vi "TestForADP.vi"() -> ()   [LabVIEW 2019]
uses:
  <vilib>/Instr/_visa.llb/VISA Configure Serial Port (Instr).vi
  <vilib>/Utility/file.llb/Write Delimited Spreadsheet (string).vi
  <vilib>/Utility/file.llb/Write Delimited Spreadsheet (DBL).vi
  <vilib>/ptbypt/NI_PtbyPt.lvlib
panel:
  out "Present (s)":dbl
  out "Elapsed Time (s)":dbl
  out "Water Warning":bool
  out "Water Alarm":bool
  out "Water Level":dbl
  out "UV Warning":bool
  out "UV Alarm":bool
  out "UV Value":dbl
  out "Lux Chart":dbl(graph)
  out "Lux Alarm":bool
  out "Lux Warning":bool
  out "Lux Value":dbl
  out "Data: Time, Humidity, Temperature, UV, Lux, Water Level":dbl[][](array[numeric])
  in  "Temp Bias":dbl
  out "Temp. Mean":dbl format="%0.2f"
  out "Temp Chart":dbl(graph)
  out "Temp Alarm":bool
  out "Temp Warning":bool
  out "Temperature (F)":dbl
  out "Humidity Chart":dbl(graph)
  out "Humid Alarm":bool
  out "Humid Warning":bool
  out "Humidity":dbl
  out "Arduino Power":bool
  in  "Operational Mode":bool
  in  "Arduino COM Port":refnum<visa-resource-name>="COM3"
  in  "?":bool
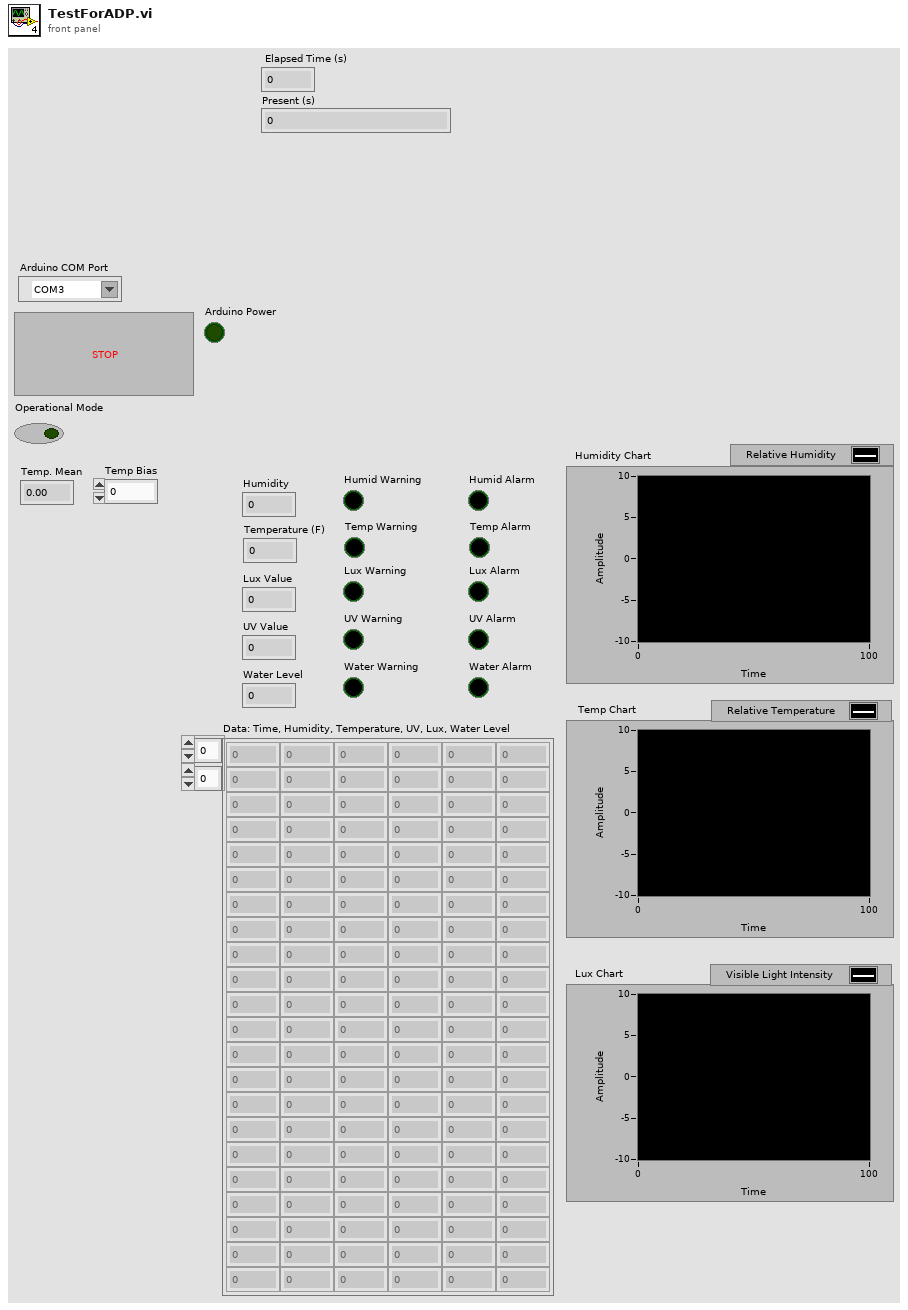
[diagram p1: front panel]
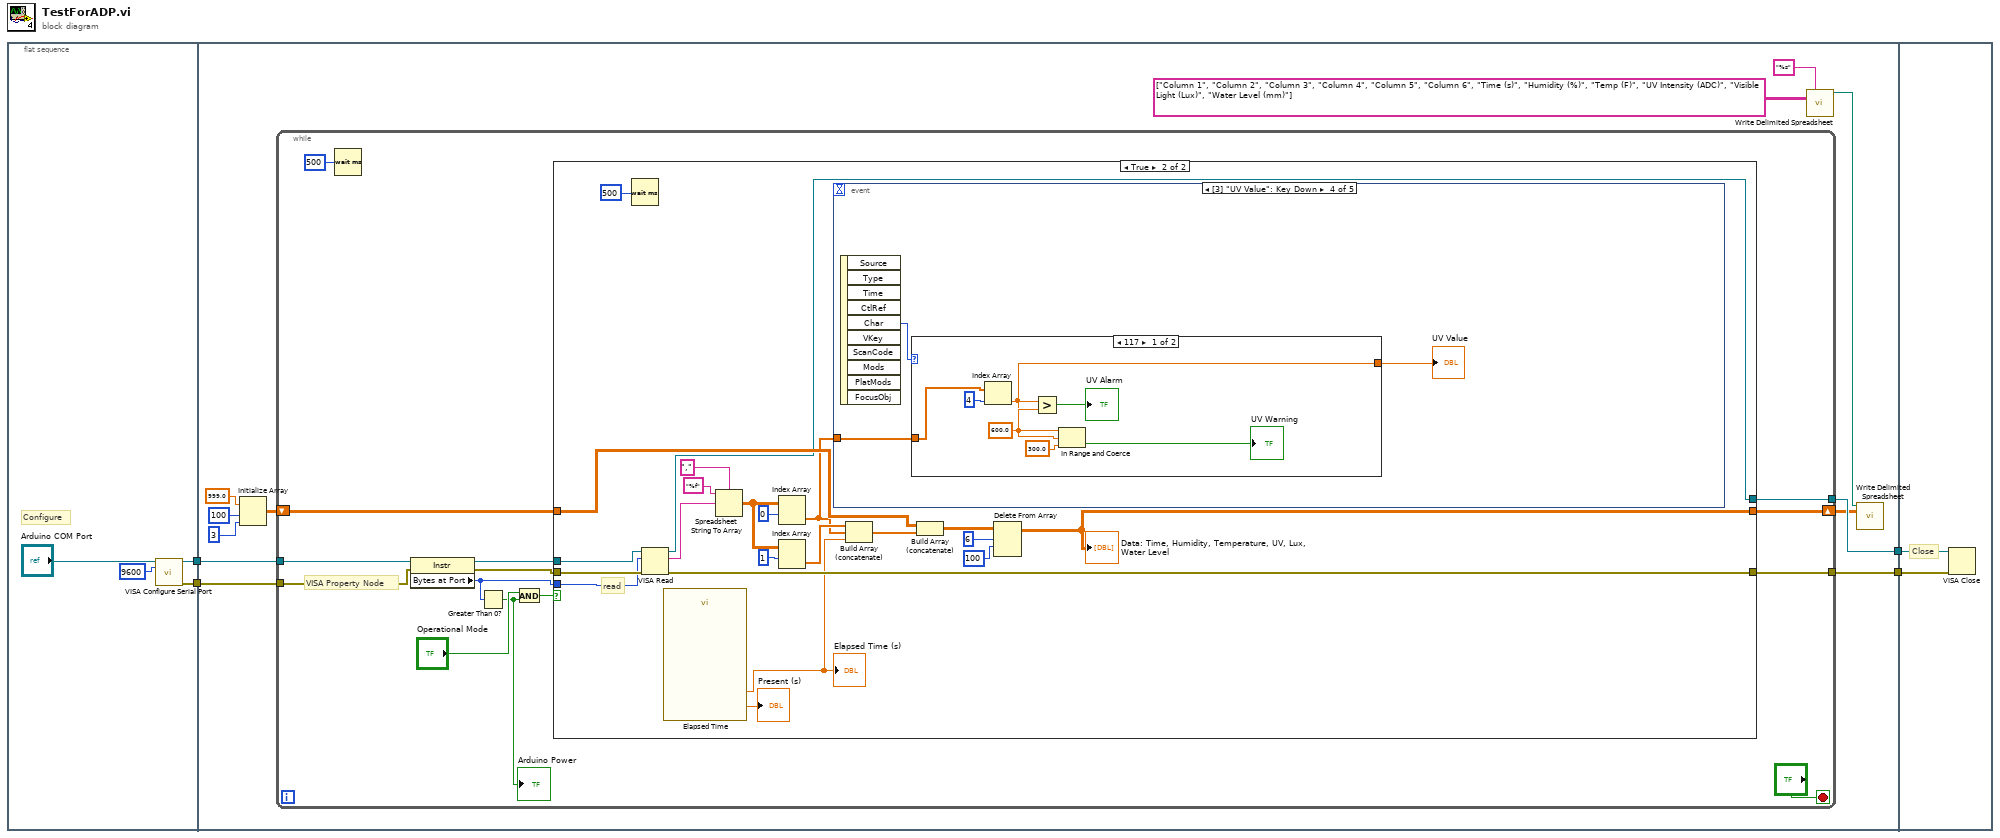
[diagram p0: block diagram]
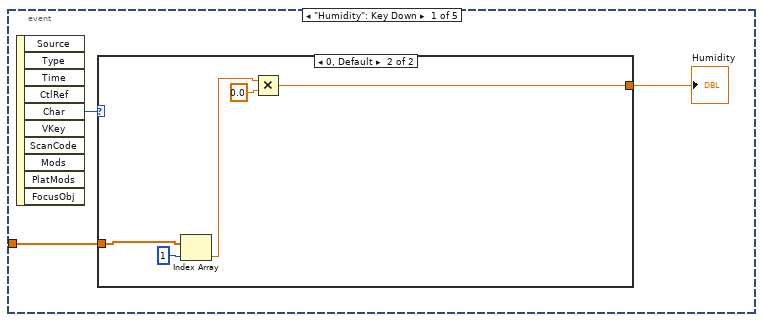
[diagram p3: hidden frame]
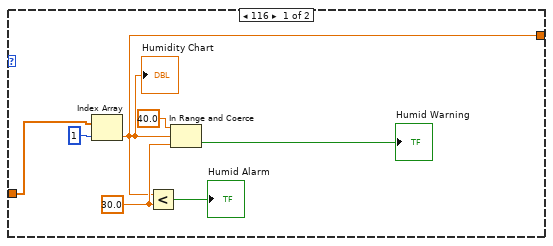
[diagram p4: hidden frame]
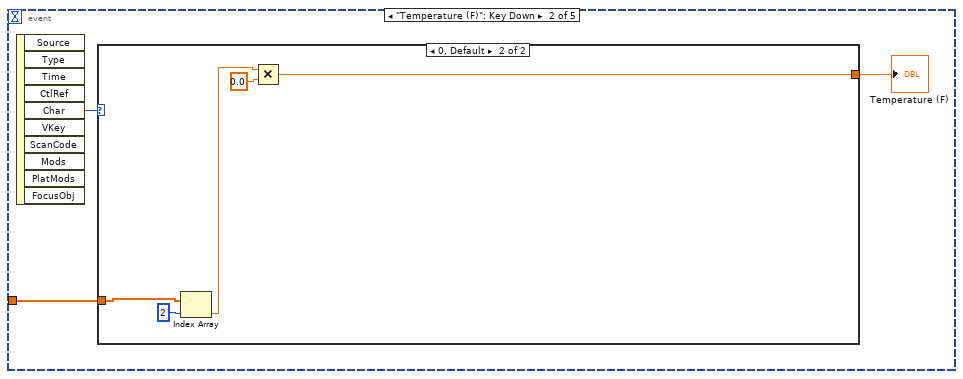
[diagram p5: hidden frame]
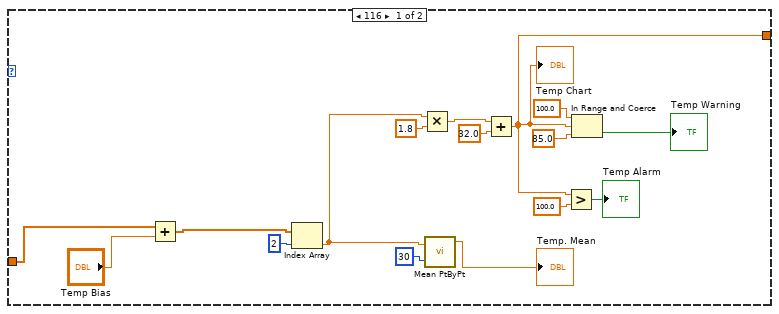
[diagram p6: hidden frame]
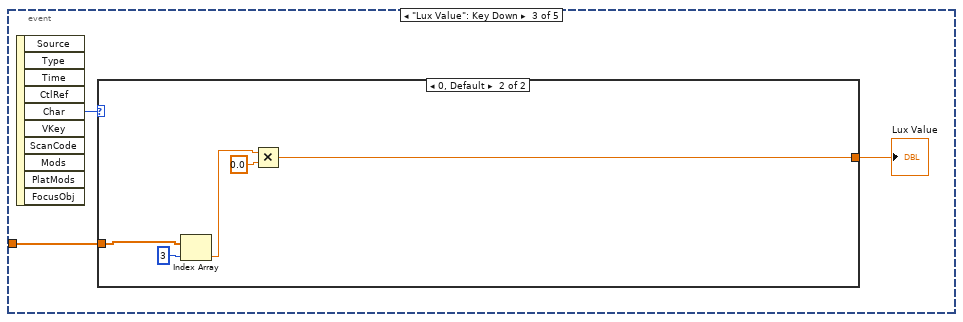
[diagram p7: hidden frame]
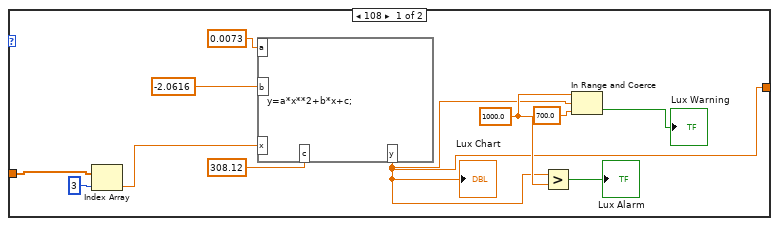
[diagram p8: hidden frame]
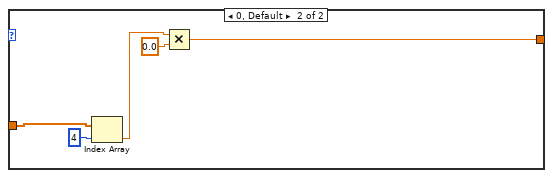
[diagram p9: hidden frame]
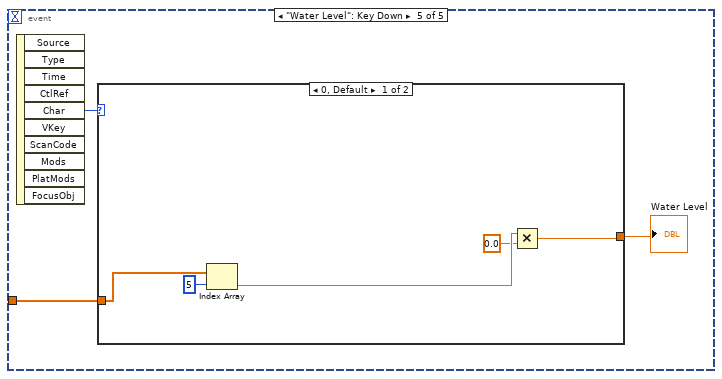
[diagram p10: hidden frame]
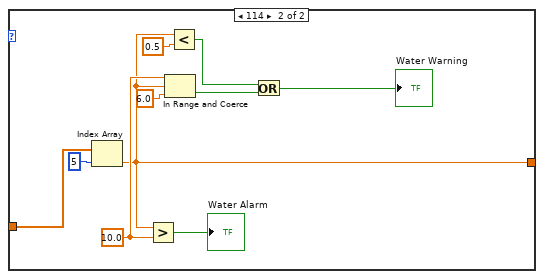
[diagram p11: hidden frame]
diagram:
  n1 = flat-sequence {
    tunnel: [w5] -> w4
    tunnel: [w6] -> w3
    tunnel: w4 -> [w20]
    tunnel: [w19] -> w2
    tunnel: w3 -> [w18]
    tunnel: [w17] -> w1
    tunnel: w2 -> [w152]
    tunnel: w1 -> [w151]
    frame #0 {
      # "Configure"
      n2 = call-poly "VISA Configure Serial Port"("VISA resource name"="Arduino COM Port", "baud rate (9600)"=u32 9600) -> ("VISA resource name out"=w5:refnum<visa-resource-name>, "error out"=w6:errorcluster)  [unwired: 12 in]
    }
    frame #1 {
      n3 = Initialize Array(999.0 ("element"), 100 ("dimension size"), 3 ("dimension size")) -> (w13:dbl[][])
      n4 = while {
        tunnel: w20 -> [w31]
        tunnel: [w23] -> w19
        tunnel: w18 -> [w30]
        tunnel: [w24] -> w17
        shift-right: [w22] -> w9
        shift-left: w13 -> [w26]
        stop <- "?" stop-if-true
        # "VISA Property Node"
        n5 = Wait (ms)(milliseconds to wait=u32 500) -> ()  [unwired: 1 out]
        n6 = property class="Instr"(reference=w31, error in=w30) -> (reference out=w28:refnum<visa-resource-name>, error out=w29:errorcluster, "Bytes at Port"=w27:u32)
        n7 = Greater Than 0?(x=w27) -> (x > 0?=w32:bool)
        "Arduino Power" <- w32
        n8 = And(x="Operational Mode", y=w32) -> (x .and. y?=w21:bool)
        n9 = case shown="True" w21 {
          tunnel: w29 -> [w36 w59]
          tunnel: w28 -> [w35 w57]
          tunnel: w27 -> [_ w58]
          tunnel: w26 -> [w37 w48]
          tunnel: [w36 w45] -> w24
          tunnel: [w35 w44] -> w23
          tunnel: [w37 w40] -> w22
          frame False {
          }
          frame True {
            # "read"
            n10 = Wait (ms)(milliseconds to wait=u32 500) -> ()  [unwired: 1 out]
            n11 = VISA Read(VISA resource name=w57, byte count=w58, error in (no error)=w59) -> (VISA resource name out=w44:refnum<visa-resource-name>, read buffer=w56:string, error out=w45:errorcluster)  [unwired: 1 out]
            n12 = call "Elapsed Time"() -> ("Present (s)"=→"Present (s)":dbl, "Elapsed Time (s)"=w39:dbl)  [unwired: 12 in, 6 out]
            "Elapsed Time (s)" <- w39
            n13 = Spreadsheet String To Array(delimiter (Tab)=",", format string="%f", spreadsheet string=w56) -> (array=w53:dbl[][])  [unwired: 1 in]
            n14 = Index Array(array=w53, index (row)=0) -> (element=w47:dbl[])  [unwired: 1 in]
            n15 = Index Array(array=w53, index (row)=1) -> (element=w50:dbl[])  [unwired: 1 in]
            n16 = event shown="[3] \"UV Value\": Key Down" {
              selector: _ -> [_ _ _ _ _]
              dyn-events: _ -> [_ _ _ _ _]
              timeout: _ -> [_ _ _ _ _]
              tunnel: w47 -> [w61 w77 w101 w120 w135]
              event "Humidity": Key Down {
                n17 = event-data() -> ("Char"=w62:i16)  [unwired: 1 in, 9 out]
                n18 = case shown="0, Default" w62 {
                  tunnel: w61 -> [w64 w73]
                  tunnel: [w63 w70] -> w60
                  frame 116 {
                    w66 = 30.0 ("y")
                    n19 = Index Array(array=w64, index=1) -> (element=w63:dbl)
                    "Humidity Chart" <- w63
                    n20 = Less?(x=w63, y=w66) -> (x < y?=→"Humid Alarm":bool)
                    n21 = In Range and Coerce(upper limit=40.0 ("y"), x=w63, lower limit=w66) -> (In Range?=→"Humid Warning":bool)  [unwired: 1 out]
                  }
                  frame 0, Default {
                    n22 = Index Array(array=w73, index=1) -> (element=w72:dbl)
                    n23 = Multiply(x=w72, y=0.0) -> (x*y=w70:dbl)
                  }
                }
                "Humidity" <- w60
              }
              event "Temperature (F)": Key Down {
                n24 = event-data() -> ("Char"=w76:i16)  [unwired: 1 in, 9 out]
                n25 = case shown="0, Default" w76 {
                  tunnel: w77 -> [w80 w97]
                  tunnel: [w78 w95] -> w75
                  frame 116 {
                    n26 = Add(x=w80, y="Temp Bias") -> (x+y=w79:dbl[])
                    n27 = Index Array(array=w79, index=2) -> (element=w82:dbl)
                    n28 = Multiply(x=w82, y=1.8) -> (x*y=w85:dbl)
                    n29 = call <vilib>:"Mean PtByPt.vi"("x"=w82, "sample length"=30) -> ("mean"=→"Temp. Mean":dbl)  [unwired: 2 in, 1 out]
                    n30 = Add(x=w85, y=32.0) -> (x+y=w78:dbl)
                    "Temp Chart" <- w78
                    n31 = Greater?(x=w78, y=100.0) -> (0:→"Temp Alarm":bool)
                    n32 = In Range and Coerce(upper limit=100.0, x=w78, lower limit=85.0 ("y")) -> (In Range?=→"Temp Warning":bool)  [unwired: 1 out]
                  }
                  frame 0, Default {
                    n33 = Index Array(array=w97, index=2) -> (element=w94:dbl)
                    n34 = Multiply(x=w94, y=0.0) -> (x*y=w95:dbl)
                  }
                }
                "Temperature (F)" <- w75
              }
              event "Lux Value": Key Down {
                n35 = event-data() -> ("Char"=w100:i16)  [unwired: 1 in, 9 out]
                n36 = case shown="0, Default" w100 {
                  tunnel: w101 -> [w104 w116]
                  tunnel: [w102 w113] -> w99
                  frame 108 {
                    w107 = 1000.0 ("y")
                    n37 = Index Array(array=w104, index=3) -> (element=w105:dbl)
                    n38 = formula code="y=a*x**2+b*x+c;"("a"=0.0073 ("input variable"), "x"=w105, "b"=-2.0616 ("input variable"), "c"=308.12 ("input variable")) -> ("y"=w102:dbl)
                    "Lux Chart" <- w102
                    n39 = Greater?(x=w102, y=w107) -> (0:→"Lux Alarm":bool)
                    n40 = In Range and Coerce(upper limit=w107, x=w102, lower limit=700.0 ("y")) -> (In Range?=→"Lux Warning":bool)  [unwired: 1 out]
                  }
                  frame 0, Default {
                    n41 = Index Array(array=w116, index=3) -> (element=w114:dbl)
                    n42 = Multiply(x=w114, y=0.0) -> (x*y=w113:dbl)
                  }
                }
                "Lux Value" <- w99
              }
              event "UV Value": Key Down {
                n43 = event-data() -> ("Char"=w119:i16)  [unwired: 1 in, 9 out]
                n44 = case shown="117" w119 {
                  tunnel: w120 -> [w123 w128]
                  tunnel: [w121 w131] -> w118
                  frame 117 {
                    w125 = 600.0 ("y")
                    n45 = Index Array(array=w123, index=4) -> (element=w121:dbl)
                    n46 = Greater?(x=w121, y=w125) -> (0:→"UV Alarm":bool)
                    n47 = In Range and Coerce(upper limit=w125, x=w121, lower limit=300.0 ("y")) -> (In Range?=→"UV Warning":bool)  [unwired: 1 out]
                  }
                  frame 0, Default {
                    n48 = Index Array(array=w128, index=4) -> (element=w129:dbl)
                    n49 = Multiply(x=w129, y=0.0) -> (x*y=w131:dbl)
                  }
                }
                "UV Value" <- w118
              }
              event "Water Level": Key Down {
                n50 = event-data() -> ("Char"=w134:i16)  [unwired: 1 in, 9 out]
                n51 = case shown="0, Default" w134 {
                  tunnel: w135 -> [w139 w142]
                  tunnel: [w136 w141] -> w133
                  frame 0, Default {
                    n52 = Index Array(array=w139, index=5) -> (element=w138:dbl)
                    n53 = Multiply(x=w138, y=0.0) -> (x*y=w136:dbl)
                  }
                  frame 114 {
                    w143 = 10.0 ("y")
                    n54 = Index Array(array=w142, index=5) -> (element=w141:dbl)
                    n55 = Greater?(x=w141, y=w143) -> (0:→"Water Alarm":bool)
                    n56 = In Range and Coerce(upper limit=w143, x=w141, lower limit=6.0 ("y")) -> (In Range?=w145:bool)  [unwired: 1 out]
                    n57 = Less?(x=w141, y=0.5) -> (x < y?=w148:bool)
                    n58 = Or(x=w148, y=w145) -> (x .or. y?=→"Water Warning":bool)
                  }
                }
                "Water Level" <- w133
              }
            }
            n59 = Build Array (concatenate)(w50, w47, w39) -> (w49:dbl[])
            n60 = Build Array (concatenate)(w48, w49) -> (w41:dbl[][])
            n61 = Delete From Array(array=w41, length=6, index (row)=100) -> (array with subset deleted=w40:dbl[][])  [unwired: 1 in, 1 out]
            "Data: Time, Humidity, Temperature, UV, Lux, Water Level" <- w40
          }
        }
      }
      n62 = call-poly <vilib>:"Write Delimited Spreadsheet.vi"("format (%s)"="%s", "2D data"=string[][] [["Column 1", "Column 2", "Column 3", "Column 4", "Column 5", "Column 6"], ["Time (s)", "Humidity (%)", "Temp (F)", "UV Intensity (ADC)", "Visible Light (Lux)", "Water Level (mm)"]]) -> ("new file path (Not A Path if cancelled)"=w10:path)  [unwired: 12 in, 1 out]
      n63 = call-poly <vilib>:"Write Delimited Spreadsheet.vi"("file path (dialog if empty)"=w10, "2D data"=w9) -> ()  [unwired: 12 in, 2 out]
    }
    frame #2 {
      # "Close"
      n64 = VISA Close(VISA resource name=w152, error in (no error)=w151) -> ()  [unwired: 1 out]
    }
  }
